vi "Maps-Set Size.vi"(0 "Google Maps Resource Out in":T1, 7 "Size":cluster{"Width":i32, "Height":i32}, 11 "error in (no error)":errorcluster) -> (4 "Google Maps Resource Out out":T1, 15 "error out":errorcluster)   [LabVIEW 2020]
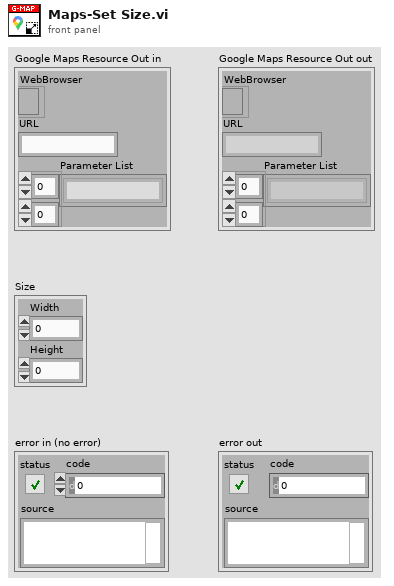
[diagram p1: front panel]
types:
  T1 = cluster{"WebBrowser":refnum<k7>, "URL":string, "Parameter List":string[][]}
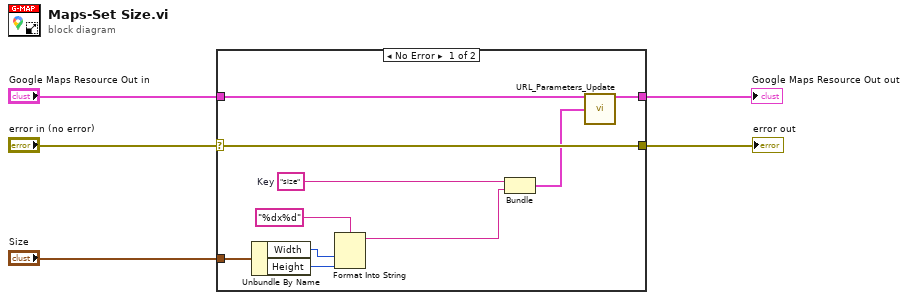
[diagram p0: block diagram]
diagram:
  n1 = case shown="No Error" "error in (no error)" {
    selector: "error in (no error)" -> [w15 w16]
    tunnel: "Google Maps Resource Out in" -> [w13 w17]
    tunnel: [w11 w17] -> w2
    tunnel: [w15 w16] -> w4
    tunnel: "Size" -> [w6 _]
    frame No Error {
      w14 = "size"  # Key
      n2 = Unbundle By Name(w6) -> ("Width"=w8:i32, "Height"=w7:i32)
      n3 = Format Into String(format string="%dx%d", w8, w7) -> (resulting string=w9:string)  [unwired: 2 in, 1 out]
      n4 = Bundle("Key"=w14, w9) -> (w12:cluster{"Key":string, string})  [unwired: 1 in]
      n5 = call "URL_Parameters_Update.vi"("Google Maps Resource In"=w13, "URL Parameter"=w12) -> ("Google Maps Resource Out"=w11:T1)  [unwired: 13 in]
    }
    frame Error {
    }
  }
  "error out" <- w4
  "Google Maps Resource Out out" <- w2
